vi "Set Multiple Object Items.vi"(5 "Item Names":string[](array[string]), 6 "$Path or Item Name":string caption="Object $Path or Item Name", 7 "error in (no error)":errorcluster, 8 "JSON Items":string[](array[string]), 9 "Object Offset":i32, 10 "JSON":string="{}") -> (0 "error out":errorcluster, 3 "<JSON>":string)   [LabVIEW 2017, in "JSONtext.lvlib"]
doc: "Insert (or replace) multiple items into a JSON Object specified by the Object $Path. \n\nIf the path specified does not exist, but its immediate parent does, then a new object is created."
uses:
  JSONtext.lvlib
  support/quote and escape json string 2.vi
  <vilib>/JDP Science/JDP Science Common Utilities/JDP Utility.lvlib
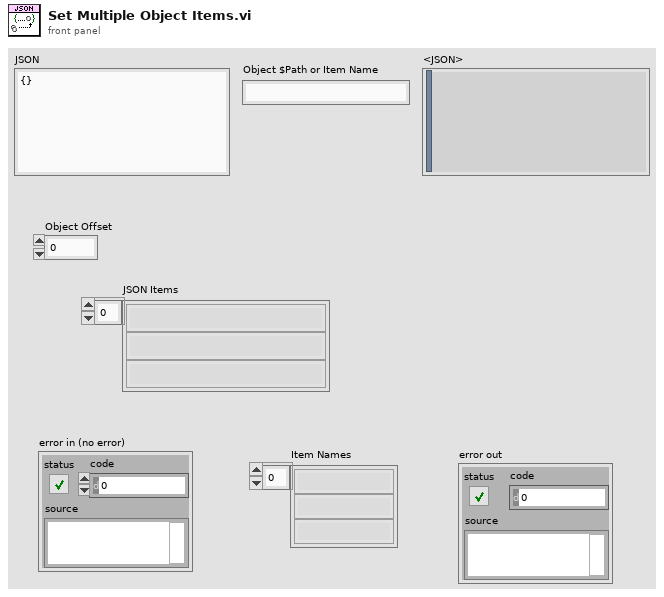
[diagram p1: front panel]
types:
  T1 = typedef "JSONtext.lvlib/Found Items.ctl" = cluster{"Item offset":i32, "Offset past Item":i32, "Name offset":i32, "Offset past Name":i32, "Found":bool, "Item Type":T2, "Item Index":i32}
  T2 = typedef "JSONtext.lvlib/Parsing State.ctl" = enum16{"Parser Error", "Object", "Array", "String", "Number/Other", "Leading Whitespace", "Object end", "Array end", "Value end"}
  T3 = cluster{"Item":T1, "<JSON>":string, "<JSON>":string}
  T4 = cluster{"Item":T1, "<JSON>":string, "<JSON>":string}[]
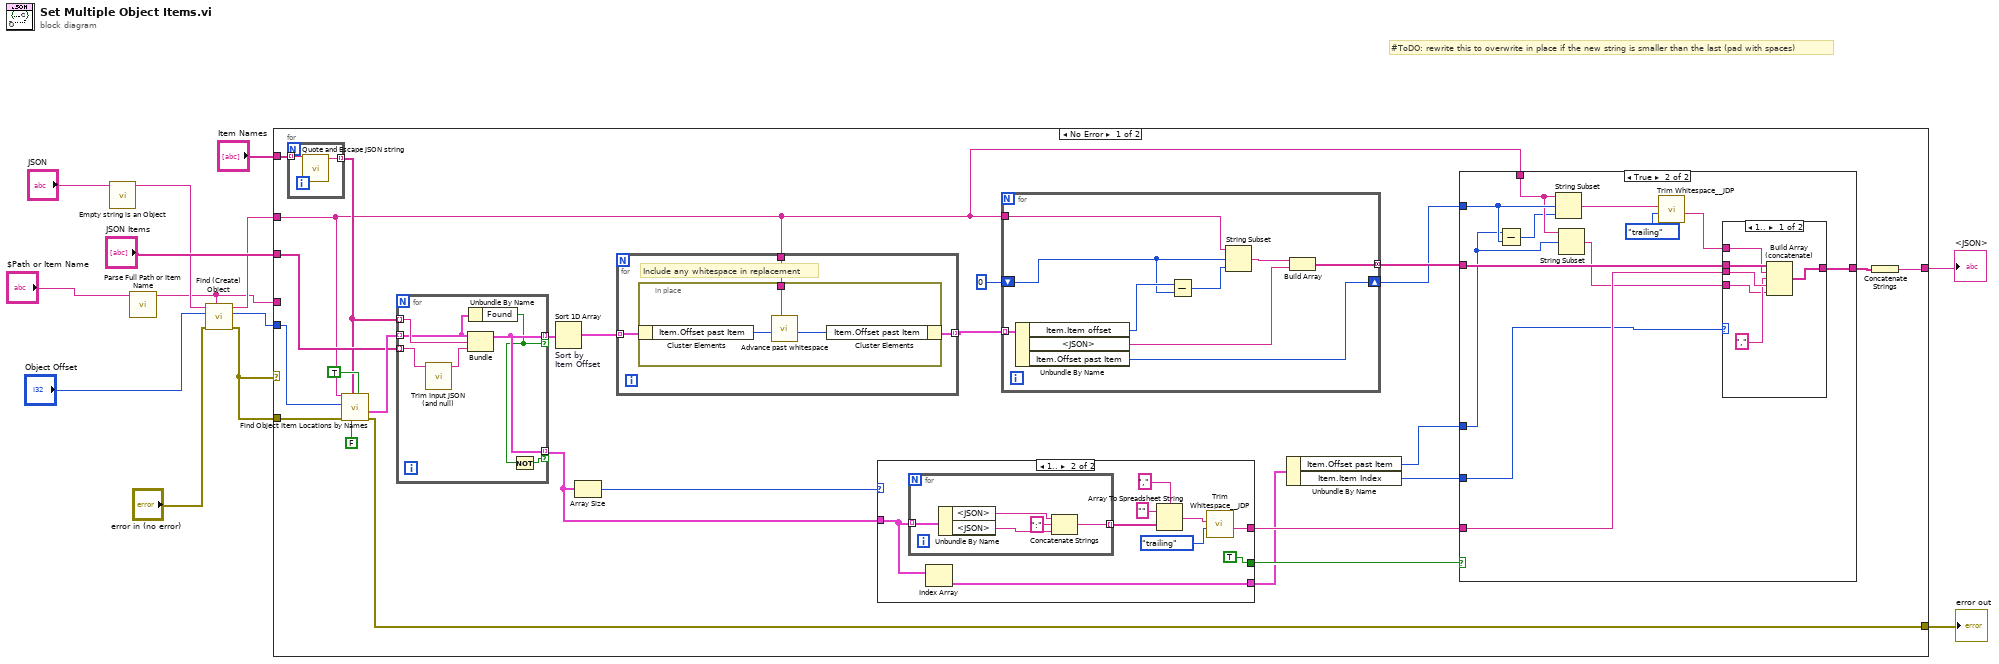
[diagram p0: block diagram]
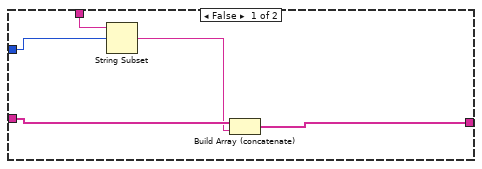
[diagram p2: hidden frame]
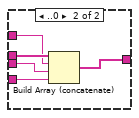
[diagram p3: hidden frame]
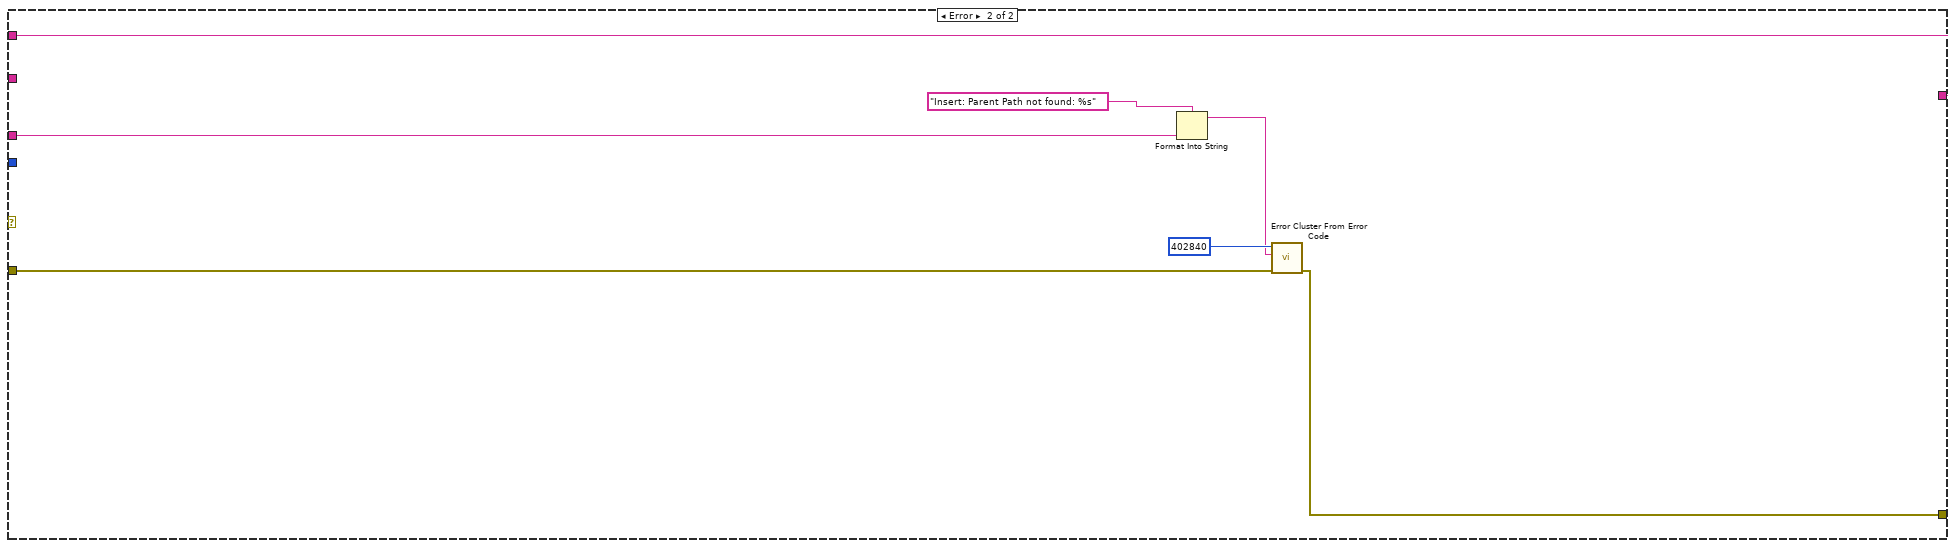
[diagram p5: hidden frame]
diagram:
  # "#ToDO: rewrite this to overwrite in place if the new string is smaller than the last (pad with spaces)"
  n1 = call "Empty string is an Object.vi"("JSON Input"="JSON") -> ("<JSON>Object"=w3:string)  [unwired: 10 in]
  n2 = call "Parse Full Path or Item Name.vi"("Full Path (with $) or Name"="$Path or Item Name") -> ("Relative Path or JSON-format name"=w2:string)  [unwired: 10 in]
  n3 = call "Find (Create) Object.vi"("Object Path"=w2, "error in (no error)"="error in (no error)", "Starting Offset"="Object Offset", "JSON"=w3) -> ("error out"=w5:errorcluster, "Object offset"=w11:i32, "<JSON>"=w7:string)  [unwired: 5 in]
  n4 = case shown="No Error" w5 {
    tunnel: "JSON Items" -> [w29 _]
    tunnel: w5 -> [w38 w105]
    tunnel: [w37 w110] -> w13
    tunnel: w7 -> [w14 w111]
    tunnel: w11 -> [w36 _]
    tunnel: "Item Names" -> [w35 _]
    tunnel: [w21 w111] -> w8
    tunnel: w2 -> [_ w106]
    frame No Error {
      n5 = for {
        tunnel: w35 -> [w104] mode=indexing
        tunnel: [w103] -> w27 mode=indexing
        n6 = call "Quote and Escape JSON string.vi"("Plain Text"=w104) -> ("<JSON>"=w103:string)  [unwired: 10 in]
      }
      n7 = call "Find Object Item Locations by Names.vi"("Insertion point if not found"=TRUE, "Only return first found"=FALSE, "Item Names <JSON>"=w27, "error in (no error)"=w38, "Object Offset"=w36, "JSON"=w14) -> ("error out"=w37:errorcluster, "Items"=w31:T1[])  [unwired: 4 in]
      n8 = for {
        tunnel: [w100] -> w32 mode=indexing if=w98
        tunnel: w31 -> [w101] mode=indexing
        tunnel: w27 -> [w102] mode=indexing
        tunnel: w29 -> [w97] mode=indexing
        tunnel: [w100] -> w26 mode=indexing if=w99
        n9 = call "Trim Input JSON (and null).vi"("JSON Input"=w97) -> ("<JSON>"=w96:string)  [unwired: 10 in]
        n10 = Bundle("Item"=w101, "<JSON>"=w102, "<JSON>"=w96) -> (w100:T3)  [unwired: 1 in]
        n11 = Unbundle By Name(w101) -> ("Found"=w98:bool)
        n12 = Not(x=w98) -> (.not. x?=w99:bool)
      }
      n13 = Sort 1D Array "Sort by \nItem Offset"(array=w32) -> (sorted array=w30:T4)
      n14 = Array Size(array=w26) -> (size(s)=w25:i32)
      n15 = for {
        tunnel: w30 -> [w83] mode=indexing
        tunnel: [w82] -> w28 mode=indexing
        tunnel: w14 -> [w81]
        # "Include any whitespace in replacement"
        n16 = in-place {
          in-place-border: w81 -> [w85]
          n17 = in-place-cluster #1(w83) -> ("Item.Offset past Item"=w86:i32)
          n18 = call "Advance past whitespace.vi"("JSON"=w85, "Offset"=w86) -> ("Offset of first non-whitespace"=w84:i32)  [unwired: 8 in, 1 out]
          n19 = in-place-cluster #1("Item.Offset past Item"=w84) -> (w82:T3)
        }
      }
      n20 = case shown="1.." w25 {
        tunnel: w26 -> [_ w70]
        tunnel: [_ w69] -> w18
        tunnel: [_ w68] -> w22
        tunnel: [_ TRUE] -> w24
        frame 0, Default {
        }
        frame 1.. {
          n21 = for {
            tunnel: w70 -> [w80] mode=indexing
            tunnel: [w76] -> w75 mode=indexing
            n22 = Unbundle By Name(w80) -> ("<JSON>"=w79:string, "<JSON>"=w78:string)
            n23 = Concatenate Strings(w79, ":" ("string"), w78) -> (w76:string)
          }
          n24 = Index Array(array=w70) -> (element=w69:T3)  [unwired: 1 in]
          n25 = Array To Spreadsheet String(delimiter (Tab)=",", array=w75, 3:"" ("format string")) -> (spreadsheet string=w72:string)
          n26 = call <vilib>:"Trim Whitespace__JDP.vi"("Remove (leading and trailing)"=enum16{"leading", "trailing", "both"}."trailing", "String in"=w72) -> ("String out"=w68:string)  [unwired: 5 in]
        }
      }
      n27 = for {
        tunnel: w14 -> [w93]
        tunnel: w28 -> [w95] mode=indexing
        tunnel: [w91] -> w23 mode=concatenating
        shift-right: [w90] -> w19
        shift-left: 0 ("Offset\nAdjustment") -> [w88]
        n28 = Unbundle By Name(w95) -> ("Item.Item offset"=w89:i32, "<JSON>"=w92:string, "Item.Offset past Item"=w90:i32)
        n29 = Subtract(x=w89, y=w88) -> (x-y=w87:i32)
        n30 = String Subset(string=w93, offset (0)=w88, length (rest)=w87) -> (substring=w94:string)
        n31 = Build Array(w94, w92) -> (w91:string[])
      }
      n32 = Unbundle By Name(w18) -> ("Item.Offset past Item"=w16:i32, "Item.Item Index"=w17:i32)
      n33 = case shown="True" w24 {
        tunnel: w23 -> [w43 w55]
        tunnel: w22 -> [_ w53]
        tunnel: [w40 w54] -> w15
        tunnel: w14 -> [w42 w50]
        tunnel: w19 -> [w41 w51]
        tunnel: w17 -> [_ w52]
        tunnel: w16 -> [_ w47]
        frame False {
          n34 = String Subset(string=w42, offset (0)=w41) -> (substring=w39:string)  [unwired: 1 in]
          n35 = Build Array (concatenate)(w43, w39) -> (w40:string[])
        }
        frame True {
          n36 = Subtract(x=w47, y=w51) -> (x-y=w49:i32)
          n37 = String Subset(string=w50, offset (0)=w51, length (rest)=w49) -> (substring=w45:string)
          n38 = String Subset(string=w50, offset (0)=w47) -> (substring=w48:string)  [unwired: 1 in]
          n39 = call <vilib>:"Trim Whitespace__JDP.vi"("Remove (leading and trailing)"=enum16{"leading", "trailing", "both"}."trailing", "String in"=w45) -> ("String out"=w44:string)  [unwired: 5 in]
          n40 = case shown="1.." w52 {
            tunnel: w55 -> [w61 w66]
            tunnel: w53 -> [w60 w65]
            tunnel: [w59 w64] -> w54
            tunnel: w44 -> [w56 w62]
            tunnel: w48 -> [w57 w63]
            frame 1.. {
              n41 = Build Array (concatenate)(w61, w56, "," ("element"), w60, w57) -> (w59:string[])
            }
            frame ..0 {
              n42 = Build Array (concatenate)(w66, w62, w65, w63) -> (w64:string[])
            }
          }
        }
      }
      n43 = Concatenate Strings(w15) -> (w21:string)
    }
    frame Error {
      n44 = Format Into String(format string="Insert: Parent Path not found: %s" ("error message (\"\")"), w106) -> (resulting string=w108:string)  [unwired: 2 in, 1 out]
      n45 = call <vilib>:"Error Cluster From Error Code.vi"("error in (no error)"=w105, "error message (\"\")"=w108, "error code (0)"=402840) -> ("error out"=w110:errorcluster)  [unwired: 6 in]
    }
  }
  "<JSON>" <- w8
  "error out" <- w13
